vi "u32.le.vi"(8 "end":u8=19, 9 "start":u8=15, 10 "Data":u8, 11 "Counter":u8) -> (3 "Latched\nValue":u32)   [LabVIEW 2022 SP3]
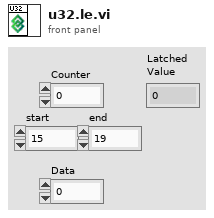
[diagram p1: front panel]
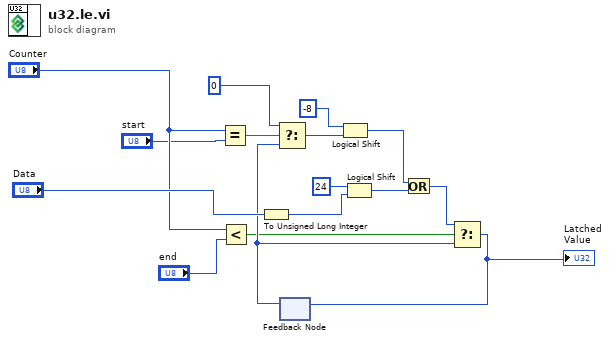
[diagram p0: block diagram]
diagram:
  n1 = Equal?(x="Counter", y="start") -> (x = y?=w3:bool)
  n2 = Less?(x="Counter", y="end") -> (x < y?=w5:bool)
  n3 = To Unsigned Long Integer(number="Data") -> (unsigned 32bit integer=w10:u32)
  n4 = feedback #1() -> (w8:u32)  [unwired: 1 in]
  n5 = Select(t=u32 0 ("y"), s=w3, f=w8) -> (s? t:f=w12:u32)
  n6 = Logical Shift(y=i16 -8, x=w12) -> (x << y=w15:u32)
  n7 = Logical Shift(y=i16 24, x=w10) -> (x << y=w11:u32)
  n8 = Or(x=w15, y=w11) -> (x .or. y?=w13:u32)
  n9 = Select(t=w13, s=w5, f=w8) -> (s? t:f=w14:u32)
  "Latched\nValue" <- w14
  n10 = feedback-in #1(w14) -> ()
